vi "CryotempCalPath.vi"() -> (0 "CryoPath":T1=path "Z:/Data/Calibration/Cryo Temp/CryoTemp.csv")   [LabVIEW 2014]
doc: "This VI defines a hardcoded path constant that is used in the init, MDS+ load and restore default settings.\n\nTo change the hardcode, type in the new path and right-click, select data operations, make current value default and save the VI."
uses:
  CryotempCalPath.ctl
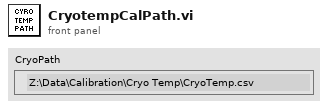
[diagram p1: front panel]
types:
  T1 = typedef "CryotempCalPath.ctl" = path
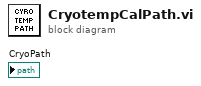
[diagram p0: block diagram]
diagram:
